vi "CheckBlackImage.vi"(8 "error in":errorcluster, 11 "Image In":T1) -> (0 "error out":errorcluster, 2 "Black?":bool, 3 "Image Out":T1)   [LabVIEW 2015]
doc: "Checks if the input image is purely black."
uses:
  <vilib>/vision/Image Controls.llb/IMAQ Image.ctl
  <vilib>/vision/NI_Vision_Development_Module.lvlib
panel:
  out "Match Flag (CheckBlackImage)":bool[](array[boolean])
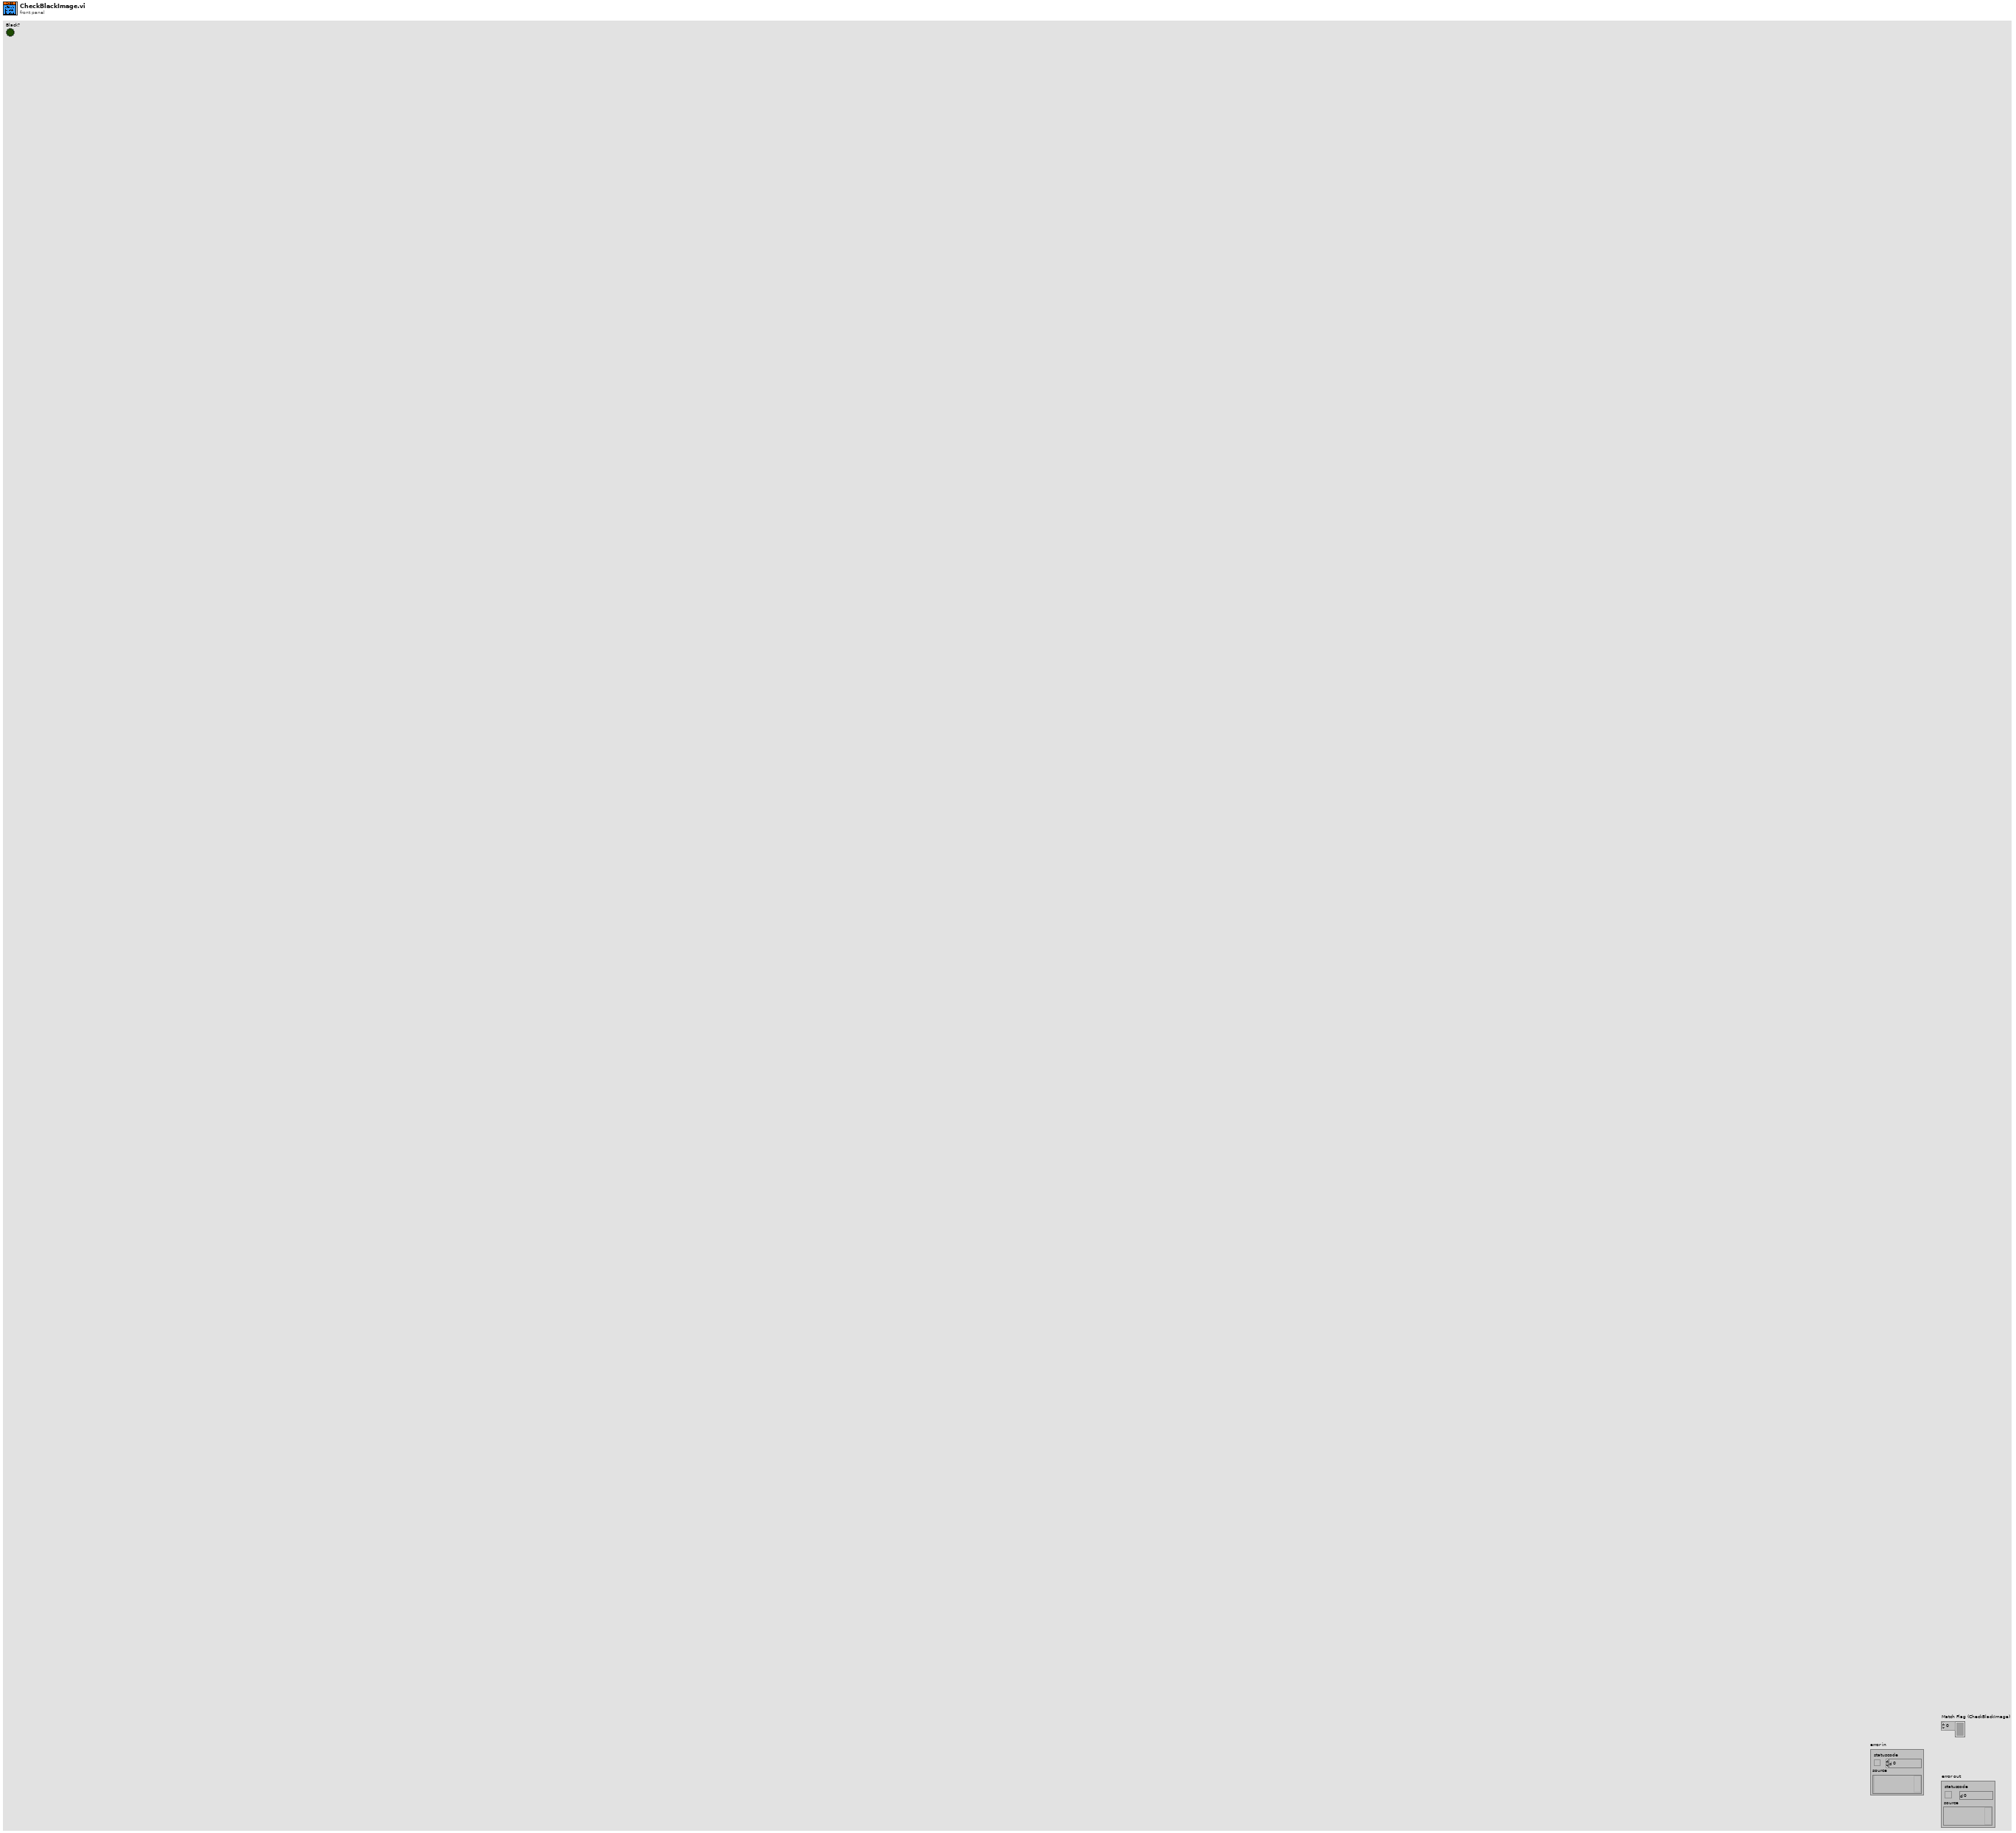
[diagram p1: front panel]
types:
  T1 = typedef "IMAQ Image.ctl" = refnum<image>
  T2 = cluster{"Global Rectangle":i32[], "Contours":cluster{"ID":enum32{"External", "Internal"}, "Type":u32, "Coordinates":i32[]}[]}
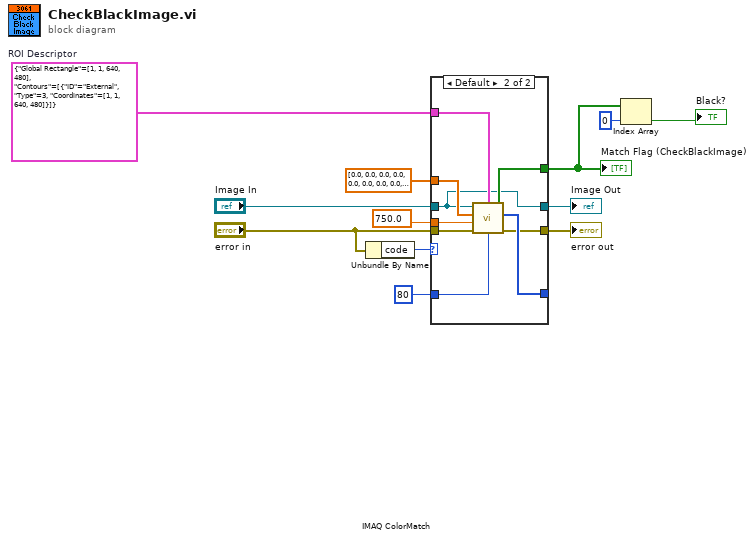
[diagram p0: block diagram]
diagram:
  w6 = T2 {"Global Rectangle"=[1, 1, 640, 480], "Contours"=[{"ID"=enum."External", "Type"=3, "Coordinates"=[1, 1, 640, 480]}]}  # ROI Descriptor
  n1 = Unbundle By Name("error in") -> ("code"=w5:i32)
  n2 = case shown="Default" w5 {
    tunnel: 750.0 ("Minimum Match Score") -> [_ w22]
    tunnel: 80 ("Match Saturation Threshold") -> [_ w21]
    tunnel: dbl[] [0.0, 0.0, 0.0, 0.0, 0.0, 0.0, 0.0, 0.0, 0.0, 0.0, 0.0, 0.0, 0.0, 0.0, 1.0, 0.0] ("Color Spectrum") -> [_ w20]
    tunnel: [_ w19] -> w1
    tunnel: [_ w18] -> _
    tunnel: "Image In" -> [w13 w14]
    tunnel: "error in" -> [_ w17]
    tunnel: [_ w16] -> w7
    tunnel: w6 -> [_ w15]
    tunnel: [w13 w14] -> w4
    frame -1074396199, -1074396198 {
      # "Discard\nCoordinate\nSystem Error"
    }
    frame Default {
      n3 = call "IMAQ ColorMatch"("ROI Descriptor"=w15, "Image"=w14, "Color Spectrum"=w20, "Match Saturation Threshold"=w21, "Minimum Match Score"=w22, "error in (no error)"=w17) -> ("Match Flag"=w19:bool[], "Match Score"=w18:i32[], "error out"=w16:errorcluster)  [unwired: 1 out]
    }
  }
  "Match Flag (CheckBlackImage)" <- w1
  "Image Out" <- w4
  "error out" <- w7
  n4 = Index Array(array=w1, index=0) -> (element=→"Black?":bool)
